vi "SwissSPAD Live_First Image.vi"(8 "error in":errorcluster) -> (0 "error out":errorcluster, 3 "Image":T1(plugin-control))   [LabVIEW 2021]
uses:
  SwissSPAD Live_Settings List.ctl
  SwissSPAD Live_Image Display Options.ctl
panel:
  in  "# Iterations":i32 format="%.0p"
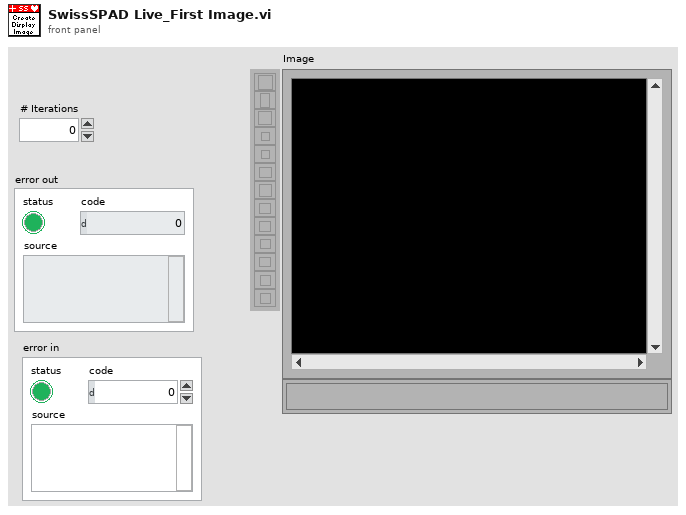
[diagram p1: front panel]
types:
  T1 = typedef "IMAQ Image.ctl" = refnum<image>
  T2 = typedef "Image Type" = u32
  T3 = typedef "SwissSPAD Live_Image Display Options.ctl" = cluster{"Remove Screamers":bool, "Delta":sgl, "Equalize Histogram":bool, "Percentile":sgl, "Hot Pixel Mask Image":path, "Use Hot Pixel Mask":bool}
  T4 = typedef "SwissSPAD Live_Settings List.ctl" = enum16{"FPGA:Bottom Half", "FPGA:Top Half", "FPGA:Bottom Bitfile Path", "FPGA:Top Bitfile Path", "FPGA:Bottom Bitstream Version", "FPGA:Top Bitstream Version", "FPGA:Auto Reset FPGA", "FPGA:Bottom FPGA Serial Number", "FPGA:Top FPGA Serial Number", "FPGA:Detector PCB Version", "Acquisition Parameters:Microlens", "Acquisition Parameters:SS2 DAQ Parameters", "Acquisition Parameters:Gate Configuration Array", "Acquisition Parameters:SS3 DAQ Parameters", "Acquisition Parameters:Buffer Size (# 8-bit Gates)", "File Information:File Information", "File Information:# Datasets in Series", "File Information:Scrambled File Flag", "File Information:SS3 Gate Slip Correction", "File Information:SS3 Hot Pixel Mismatch Detection", "File Information:Delay between Datasets", "File Information:Save Sum of All Gates Preview", "Image Parameters:Image ROI Information", "Image Parameters:Image Binning Options", "Image Parameters:SS3 Displayed Image", "Image Parameters:Image Display Options", "Image Parameters:Use Histogram Cursors", "Image Parameter:FPGA Data to Display", "UI Settings:Histogram Bins Number", "UI Settings:Histogram Bin Size", "UI Settings:Use Image Display Options", "UI Settings:Verbose Settings", "UI Settings:Verbose Saving"}
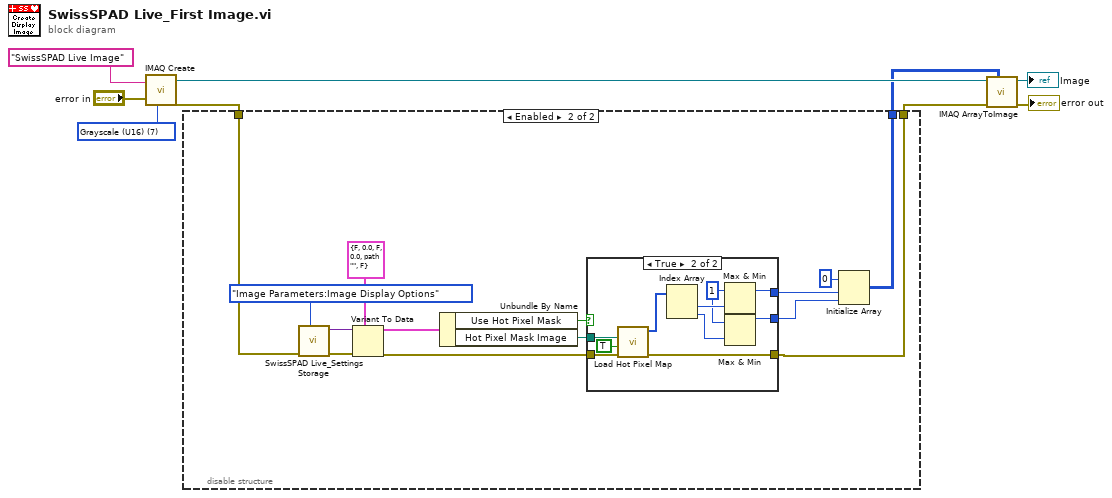
[diagram p0: block diagram]
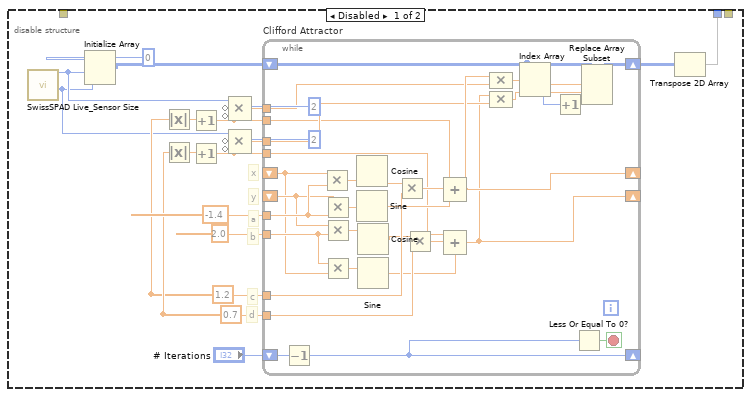
[diagram p2: hidden frame]
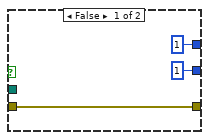
[diagram p3: hidden frame]
diagram:
  w9 = T2 7 items=["Grayscale (U8)", "Grayscale (I16)", "Grayscale (SGL)", "Complex (CSG)", "RGB (U32)", "HSL (U32)", "RGB (U64)", "Grayscale (U16)"] ("Image Type")
  n1 = call "IMAQ Create"("Image Name"="SwissSPAD Live Image", "Image Type"=w9, "error in (no error)"="error in") -> ("New Image"=w5:T1, "error out"=w3:errorcluster)  [unwired: 2 in]
  n2 = disable-structure shown="Enabled" {
    disable-tunnel: [w10 w67] -> w4
    disable-tunnel: w3 -> [_ w73]
    disable-tunnel: [_ w62] -> w2
    frame Disabled {
      w16 = 0.7
      w15 = 1.2
      # "d"
      # "c"
      # "b"
      # "a"
      # "y"
      # "x"
      n3 = call "SwissSPAD Live_Sensor Size.vi"() -> ("Y size"=w11:i32, "X size"=w12:i32)  [unwired: 9 in, 1 out]
      n4 = Initialize Array(u16 0 ("element"), w12, w11) -> (w14:u16[][])
      n5 = Absolute Value(x=w15) -> (abs(x)=w26:dbl)
      n6 = Absolute Value(x=w16) -> (abs(x)=w22:dbl)
      n7 = Increment(x=w26) -> (x+1=w20:dbl)
      n8 = Increment(x=w22) -> (x+1=w19:dbl)
      n9 = Compound Arithmetic op=MULTIPLY(w12, invert 2 ("value"), invert w20) -> (w24:dbl)
      n10 = Compound Arithmetic op=MULTIPLY(w11, invert 2 ("value"), invert w19) -> (w21:dbl)
      n11 = while "Clifford Attractor" {
        shift-right: [w43] -> _
        shift-left: _ -> [w34]
        shift-right: [w36] -> _
        shift-left: _ -> [w35]
        tunnel: -1.4 ("Numeric") -> [w59]
        tunnel: 2.0 ("Numeric") -> [w51]
        tunnel: w15 -> [w56]
        tunnel: w16 -> [w48]
        shift-right: [w29] -> w28
        shift-left: w14 -> [w33]
        shift-right: [w30] -> _
        shift-left: "# Iterations" -> [w42]
        tunnel: w24 -> [w40]
        tunnel: w21 -> [w39]
        tunnel: w20 -> [w38]
        tunnel: w19 -> [w37]
        stop <- w41 stop-if-true
        n12 = Decrement(x=w42) -> (x-1=w30:i32)
        n13 = Multiply(x=w34, y=w59) -> (x*y=w58:dbl)
        n14 = Multiply(x=w35, y=w59) -> (x*y=w55:dbl)
        n15 = Multiply(x=w35, y=w51) -> (x*y=w52:dbl)
        n16 = Multiply(x=w51, y=w34) -> (x*y=w50:dbl)
        n17 = Cosine(x=w58) -> (cos(x)=w57:dbl)
        n18 = Sine(x=w55) -> (sin(x)=w54:dbl)
        n19 = Cosine(x=w52) -> (cos(x)=w49:dbl)
        n20 = Sine(x=w50) -> (sin(x)=w46:dbl)
        n21 = Multiply(x=w57, y=w56) -> (x*y=w53:dbl)
        n22 = Multiply(x=w49, y=w48) -> (x*y=w47:dbl)
        n23 = Compound Arithmetic op=ADD(w38, w53, w54) -> (w43:dbl)
        n24 = Compound Arithmetic op=ADD(w37, w47, w46) -> (w36:dbl)
        n25 = Compound Arithmetic op=MULTIPLY(w43, w40) -> (w32:dbl)
        n26 = Compound Arithmetic op=MULTIPLY(w36, w39) -> (w31:dbl)
        n27 = Index Array(array=w33, index (row)=w32, index (col)=w31) -> (element=w44:u16)
        n28 = Increment(x=w44) -> (x+1=w45:u16)
        n29 = Less Or Equal To 0?(x=w30) -> (x <= 0?=w41:bool)
        n30 = Replace Array Subset(array=w33, new element=w45, index (row)=w32, index (col)=w31) -> (w29:u16[][])
      }
      n31 = Transpose 2D Array(2D array=w28) -> (transposed array=w10:u16[][])
    }
    frame Enabled {
      n32 = call "SwissSPAD Live_Settings Storage.vi"("Settings List"=SwissSPAD_Live_Settings_List."Image Parameters:Image Display Options", "Error In"=w73) -> ("Error Out"=w71:errorcluster, "Variant Data out"=w72:variant)  [unwired: 8 in]
      n33 = Variant To Data(error in=w71, type=T3 {"Remove Screamers"=FALSE, "Delta"=0.0, "Equalize Histogram"=FALSE, "Percentile"=0.0, "Hot Pixel Mask Image"=path "", "Use Hot Pixel Mask"=FALSE} ("Image Display Options"), Variant=w72) -> (data=w60:T3, error out=w68:errorcluster)
      n34 = Unbundle By Name(w60) -> ("Use Hot Pixel Mask"=w65:bool, "Hot Pixel Mask Image"=w69:path)
      n35 = case shown="True" w65 {
        tunnel: w69 -> [_ w86]
        tunnel: w68 -> [w76 w85]
        tunnel: [w76 w84] -> w62
        tunnel: [1 w82] -> w64
        tunnel: [1 w78] -> w63
        frame False {
        }
        frame True {
          w80 = 1 ("x")
          n36 = call "Load Hot Pixel Map.vi"("Error In"=w85, "Verbose (F)"=TRUE, "Hot Pixel Mask Image Path"=w86) -> ("Error Out"=w84:errorcluster, "Mask Image Dimensions"=w83:i32[])  [unwired: 7 in]
          n37 = Index Array(array=w83) -> (element #1=w81:i32, element #2=w79:i32)  [unwired: 2 in]
          n38 = Max & Min(x=w80, y=w81) -> (max(x,y)=w82:i32)  [unwired: 1 out]
          n39 = Max & Min(x=w80, y=w79) -> (max(x,y)=w78:i32)  [unwired: 1 out]
        }
      }
      n40 = Initialize Array(u16 0, w64, w63) -> (w67:u16[][])
    }
  }
  n41 = call "IMAQ ArrayToImage"("Image Pixels (U16)"=w4, "error in (no error)"=w2, "Image"=w5) -> ("error out"=→"error out":errorcluster, "Image Out"=→"Image":T1)  [unwired: 7 in]
